vi "Stamp interface with PWM and calibration.vi"(8 "Data Status":T2, 10 "Plant State":u16(ring)=1) -> (1 "Stamp com success":bool, 2 "Controls out 2":T1 {"fractional duty" format="%#_3g"}, 3 "Controls out 1":T1 {"fractional duty" format="%#_3g"})   [LabVIEW 2012]
uses:
  Process Controller 3.0/switch and fraction.ctl
  Process Controller 3.0/data status.ctl
  Process Controller 3.0/logic buffer cmd.ctl
  stamp command.ctl
panel:
  out "tries":i32
  in  "Controls default":T1=[{"switch"=FALSE, "fractional duty"=0.0}, {"switch"=FALSE, "fractional duty"=0.0}, {"switch"=FALSE, "fractional duty"=0.0}, {"switch"=FALSE, "fractional duty"=0.0}, {"switch"=FALSE, "fractional duty"=0.0}, {"switch"=FALSE, "fractional duty"=0.0}, {"switch"=FALSE, "fractional duty"=0.0}, {"switch"=FALSE, "fractional duty"=0.0}, {"switch"=FALSE, "fractional duty"=0.0}, {"switch"=FALSE, "fractional duty"=0.0}, {"switch"=FALSE, "fractional duty"=0.0}, {"switch"=FALSE, "fractional duty"=0.0}, {"switch"=FALSE, "fractional duty"=0.0}, {"switch"=FALSE, "fractional duty"=0.0}, {"switch"=FALSE, "fractional duty"=0.0}, {"switch"=FALSE, "fractional duty"=0.0}] {"fractional duty" format="%#_3g"}
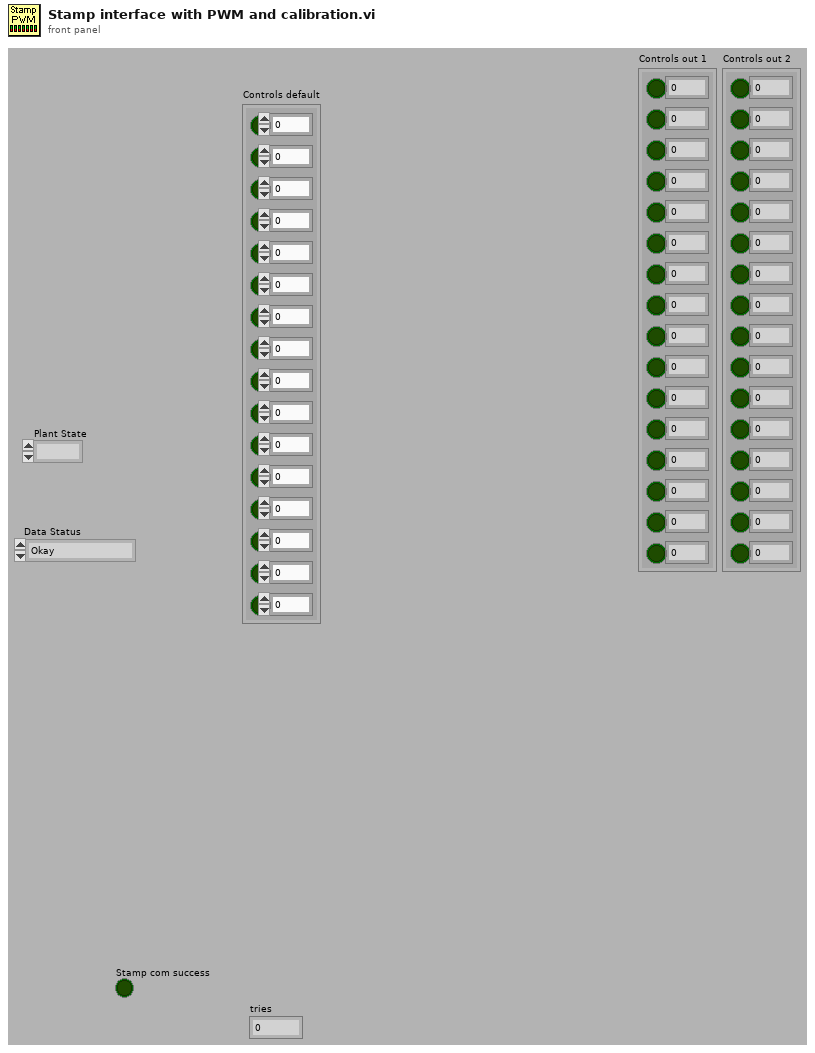
[diagram p1: front panel]
types:
  T1 = typedef "switch and fraction.ctl" = cluster{"switch":bool, "fractional duty":dbl}[]
  T2 = typedef "data status.ctl" = enum16{"Okay", "Sensor Range error", "Server error"}
  T3 = typedef "logic buffer cmd.ctl" = enum16{"read", "write ouput settings", "write rules", "write setpoints", "write output descriptions", "write all", "calculate setpoints", "save", "open", "Load all setpoint code", "Load one setpoint code", "Configure one setpoint code"}
  T4 = typedef "stamp command.ctl" = enum16{"Configure", "Write", "Off", "Close"}
  T5 = typedef "variable setpoint.ctl" = cluster{"name":string, "unit":string, "value":dbl, "Type":enum16{"Constant", "Variable"}, "variable":cluster{"selected sensors":i32[], "selected set points":i32[], "VI":path, "Data average interval":T6, "code ref":T7}}
  T6 = typedef "data ave interval.ctl" = dbl
  T7 = typedef "type specifier for control code.ctl" = refnum<vi>
  T8 = typedef "Output control.ctl" = u16[][]
  T9 = typedef "Stamp 2 control.ctl" = cluster{"Switches":bool[], "Pumps":T10[]}
  T10 = typedef "Pump w direction.ctl" = cluster{"on/off":T11, "Direction":T12, "flow rate":dbl[unit], "Tubing":T13, "tubing or 0 to 1":bool, "0 to 1":dbl}
  T11 = typedef "mini peristaltic pump.ctl" = bool
  T12 = typedef "Pump Direction.ctl" = bool
  T13 = typedef "3-stop colors and numbers.ctl" = enum16{"orange-black", "orange-red", "orange-blue", "orange-green", "green-yellow", "orange-yellow", "white-yellow", "orange-white", "black-black", "orange-orange", "white-black", "white-white", "white-red", "red-red", "red-grey", "grey-grey", "yellow-yellow", "yellow-blue", "blue-blue", "blue-green", "green-green", "purple-purple", "purple-black", "purple-orange", "purple-white", "black-white", "13", "14", "15", "16", "17", "18"}
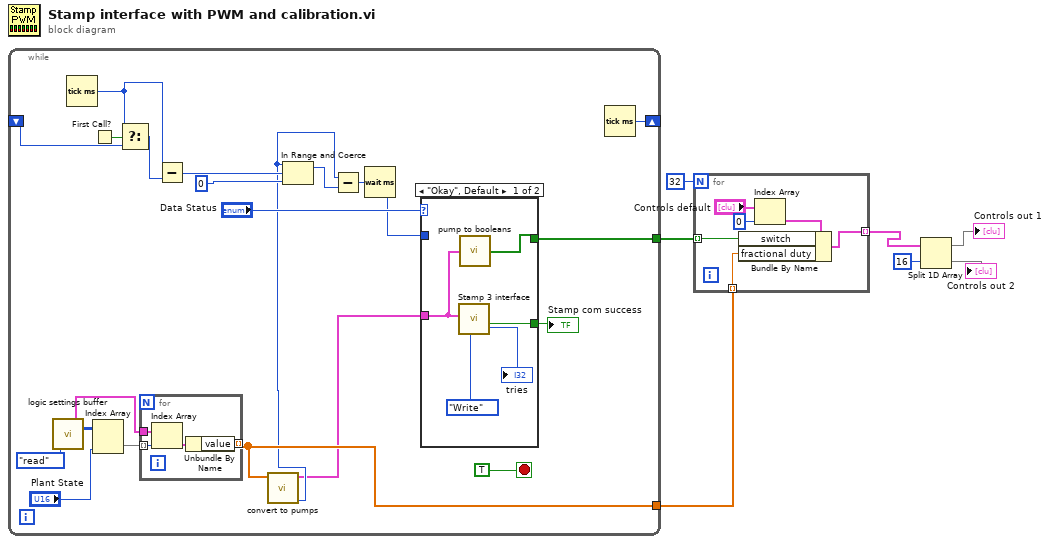
[diagram p0: block diagram]
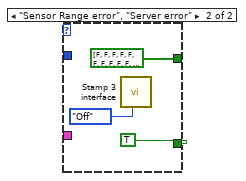
[diagram p2: hidden frame]
diagram:
  n1 = while {
    shift-right: [w20] -> _
    shift-left: _ -> [w25]
    tunnel: [w10] -> w7
    tunnel: [w18] -> w5
    stop <- TRUE stop-if-true
    n2 = call "logic settings buffer.vi"("command"=logic_buffer_cmd."read") -> ("Set Points out"=w15:T5[], "ouput settings out"=w28:T8)  [unwired: 11 in, 6 out]
    n3 = Tick Count (ms)() -> (millisecond timer value=w19:u32)
    n4 = First Call?() -> (First Call?: T/F=w26:bool)
    n5 = Index Array(array=w28, index (col)="Plant State") -> (element=w16:u16[])  [unwired: 1 in]
    n6 = Select(t=w19, s=w26, f=w25) -> (s? t:f=w24:u32)
    n7 = for {
      tunnel: w16 -> [w41] mode=indexing
      tunnel: w15 -> [w40]
      tunnel: [w38] -> w10 mode=indexing
      n8 = Index Array(array=w40, index=w41) -> (element=w39:T5)
      n9 = Unbundle By Name(w39) -> ("value"=w38:dbl)
    }
    n10 = Subtract(x=w19, y=w24) -> (x-y=w23:u32)
    n11 = call "convert to pumps.vi"("control values"=w10) -> ("minimum pulse time (ms) 2"=w9:u32, "Control out"=w8:T9)  [unwired: 9 in]
    n12 = In Range and Coerce(upper limit=w9, x=w23, lower limit=u32 0) -> (coerced(x)=w21:u32)  [unwired: 1 out]
    n13 = Subtract(x=w9, y=w21) -> (x-y=w13:u32)
    n14 = Wait (ms)(milliseconds to wait=w13) -> (millisecond timer value=w12:u32)
    n15 = case shown="\"Okay\", Default" "Data Status" {
      tunnel: [w31 bool[] [FALSE, FALSE, FALSE, FALSE, FALSE, FALSE, FALSE, FALSE, FALSE, FALSE, FALSE, FALSE, FALSE, FALSE, FALSE, FALSE, FALSE, FALSE, FALSE, FALSE, FALSE, FALSE, FALSE, FALSE, FALSE, FALSE, FALSE, FALSE, FALSE, FALSE, FALSE, FALSE] ("inverting")] -> w18
      tunnel: w12 -> [_ _]
      tunnel: [w32 TRUE ("success?")] -> w11
      tunnel: w8 -> [w30 _]
      frame "Okay", Default {
        n16 = call "Stamp 3 interface.vi"("Stamp Command"=stamp_command."Write", "Control"=w30) -> ("success?"=w32:bool, "tries"=→"tries":i32)  [unwired: 7 in, 1 out]
        n17 = call "pump to booleans.vi"("Control"=w30) -> ("controls boolean"=w31:bool[])
      }
      frame "Sensor Range error", "Server error" {
        n18 = call "Stamp 3 interface.vi"("Stamp Command"=stamp_command."Off") -> ()  [unwired: 8 in, 3 out]
      }
    }
    "Stamp com success" <- w11
    n19 = Tick Count (ms)() -> (millisecond timer value=w20:u32)
  }
  n20 = for {
    N: 32 -> [_]
    tunnel: w5 -> [w47] mode=indexing
    tunnel: w7 -> [w46] mode=indexing
    tunnel: [w45] -> w4 mode=indexing
    n21 = Index Array(array="Controls default", index=0) -> (element=w42:cluster{"switch":bool, "fractional duty":dbl})
    n22 = Bundle By Name(cluster=w42, "switch"=w47, "fractional duty"=w46) -> (w45:cluster{"switch":bool, "fractional duty":dbl})
  }
  n23 = Split 1D Array(array=w4, index=16) -> (first subarray=→"Controls out 1":cluster{"switch":bool, "fractional duty":dbl}[], second subarray=→"Controls out 2":cluster{"switch":bool, "fractional duty":dbl}[])
